vi "Sort spreadsheet.vi"(8 "error in (no error)":errorcluster, 9 "Descending (F)":bool, 10 "Priority Columns (0)":i32[](array[numeric])=[0], 11 "Unsorted Spreadsheet":string[][](array[string])) -> (0 "error out":errorcluster, 3 "Sorted Spreadsheet":string[][](array[string]))   [LabVIEW 2013]
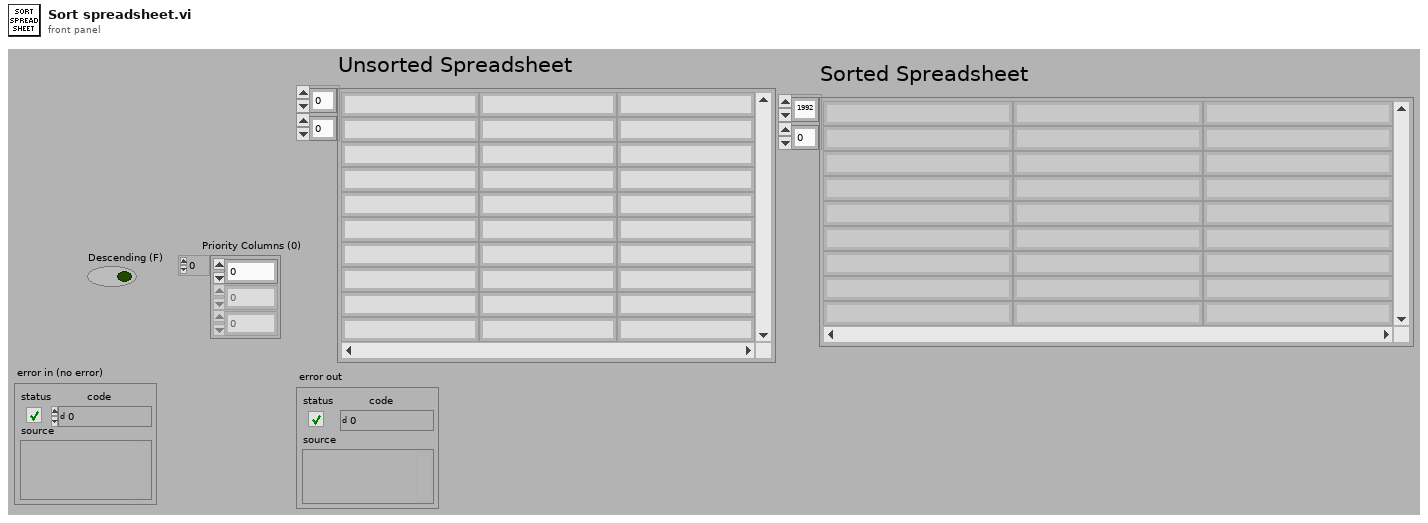
[diagram p1: front panel]
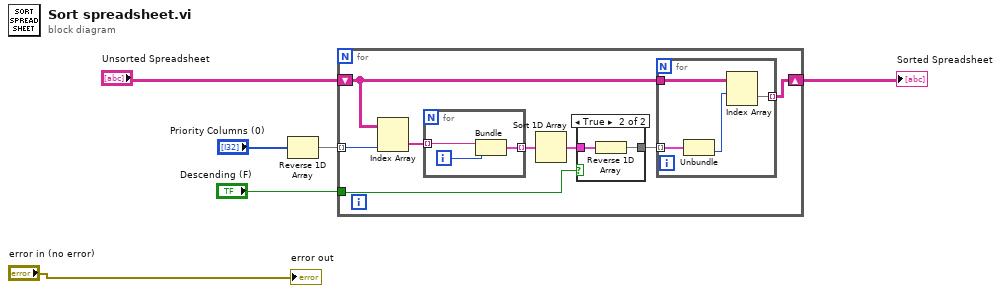
[diagram p0: block diagram]
diagram:
  n1 = Reverse 1D Array(array="Priority Columns (0)") -> (reversed array=w5:i32[])
  n2 = for {
    shift-right: [w8] -> w1
    shift-left: "Unsorted Spreadsheet" -> [w10]
    tunnel: w5 -> [w7] mode=indexing
    tunnel: "Descending (F)" -> [w9]
    n3 = Index Array(array=w10, index (col)=w7) -> (element=w12:string[])  [unwired: 1 in]
    n4 = for {
      tunnel: w12 -> [w22] mode=indexing
      tunnel: [w24] -> w11 mode=indexing
      i -> [w23]
      n5 = Bundle("String"=w22, w23) -> (w24:cluster{"String":string, i32})  [unwired: 1 out]
    }
    n6 = Sort 1D Array(array=w11) -> (sorted array=w14:cluster{"String":string, i32}[])
    n7 = case shown="True" w9 {
      tunnel: [w15 w16] -> w13
      tunnel: w14 -> [w15 w17]
      frame False {
      }
      frame True {
        n8 = Reverse 1D Array(array=w17) -> (reversed array=w16:cluster{"String":string, i32}[])
      }
    }
    n9 = for {
      tunnel: w13 -> [w21] mode=indexing
      tunnel: w10 -> [w20]
      tunnel: [w18] -> w8 mode=indexing
      n10 = Unbundle(w21) -> (w19:i32)  [unwired: 1 out]
      n11 = Index Array(array=w20, index (row)=w19) -> (element=w18:string[])  [unwired: 1 in]
    }
  }
  "Sorted Spreadsheet" <- w1
  "error out" <- "error in (no error)"
